vi "Gif.ImageData.vi"(0 "data":string, 9 "offset":i32, 11 "error in (no error)":errorcluster, 12 "ImageDescriptor":T1) -> (4 "data out":string, 6 "Index Array":i32[](array[numeric]), 10 "offset out":i32, 15 "error out":errorcluster)   [LabVIEW 2011]
uses:
  Gif.ImageDescriptor.ctl
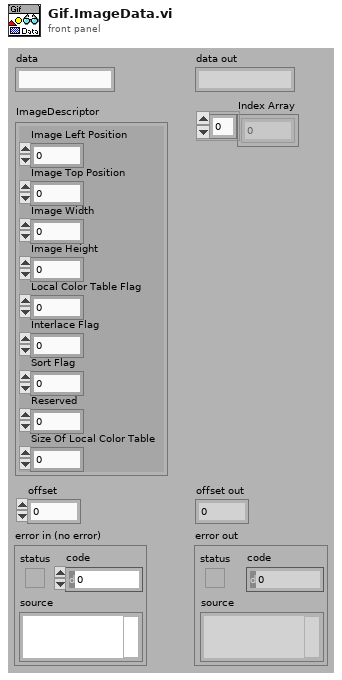
[diagram p1: front panel]
types:
  T1 = typedef "Gif.ImageDescriptor.ctl" = cluster{"Image Left Position":u16, "Image Top Position":u16, "Image Width":u16, "Image Height":u16, "Local Color Table Flag":u8, "Interlace Flag":u8, "Sort Flag":u8, "Reserved":u8, "Size Of Local Color Table":u8}
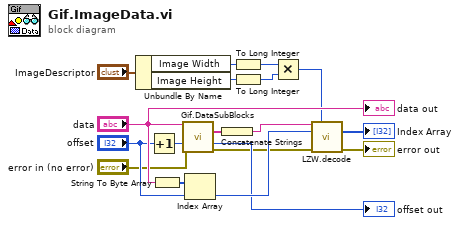
[diagram p0: block diagram]
diagram:
  n1 = Unbundle By Name("ImageDescriptor") -> ("Image Width"=w5:u16, "Image Height"=w3:u16)
  n2 = Increment(x="offset") -> (x+1=w15:i32)
  n3 = String To Byte Array(string="data") -> (unsigned byte array=w18:u8[])
  n4 = call "Gif.DataSubBlocks.vi"("data"="data", "offset"=w15, "error in (no error)"="error in (no error)") -> ("SubBlock values"=w13:string[], "offset out"=→"offset out":i32, "error out"=w9:errorcluster)  [unwired: 10 out]
  n5 = Index Array(array=w18, index="offset") -> (element=w17:u8)
  n6 = Concatenate Strings(w13) -> (w12:string)
  n7 = To Long Integer(number=w5) -> (32bit integer=w2:i32)
  n8 = To Long Integer(number=w3) -> (32bit integer=w1:i32)
  n9 = Multiply(x=w2, y=w1) -> (x*y=w4:i32)
  n10 = call "LZW.decode.vi"("data"=w12, "expected data size"=w4, "NumberOfStartBits"=w17, "error in (no error)"=w9) -> ("decoded data"=→"Index Array":i32[], "error out"=→"error out":errorcluster)  [unwired: 10 out]
  "data out" <- "data"
